vi "IO_Number of spectra Samples.vi"(10 "cor":T1) -> (2 "number of samples":i32)   [LabVIEW 2011]
doc: "Returns the number of data elements in the waveform. You must manually select the polymorphic instance you want to use."
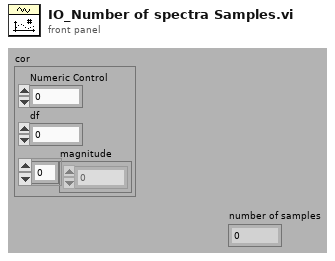
[diagram p1: front panel]
types:
  T1 = cluster{"Numeric Control":dbl, "df":dbl, "magnitude":dbl[]}
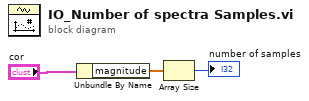
[diagram p0: block diagram]
diagram:
  n1 = Unbundle By Name("cor") -> ("magnitude"=w1:dbl[])
  n2 = Array Size(array=w1) -> (size(s)=→"number of samples":i32)
